vi "PicoErrorHandler.vi"(1 "error in":errorcluster) -> (0 "error out":errorcluster)   [LabVIEW 2020]
doc: "This VI takes an error cluster and if an error has occurred, displays a message box indicating the source of the error and the status code returned by the driver."
uses:
  DialogType.ctl
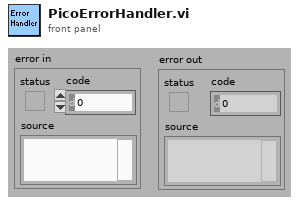
[diagram p1: front panel]
types:
  T1 = typedef "DialogType.ctl" = u16
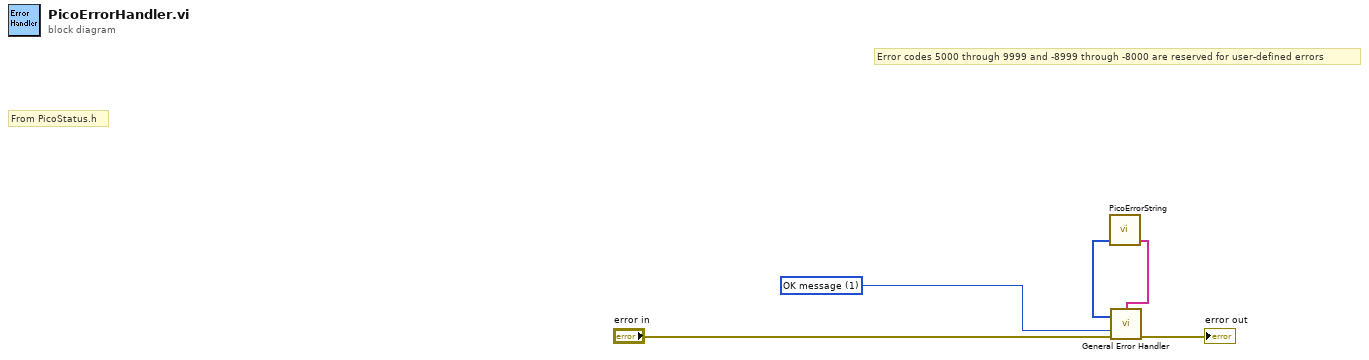
[diagram p0: block diagram]
diagram:
  w5 = T1 1 items=["no dialog", "OK message", "continue or stop message", "OK message + warnings", "continue/stop + warnings"] ("type of dialog (OK msg:1)")
  # "Error codes 5000 through 9999 and -8999 through -8000 are reserved for user-defined errors"
  # "From PicoStatus.h"
  n1 = call "PicoErrorString.vi"() -> ("[user-defined descriptions]"=w1:string[], "[user-defined codes]"=w2:u32[])  [unwired: 3 in, 1 out]
  n2 = call "General Error Handler.vi"("[user-defined codes]"=w2, "[user-defined descriptions]"=w1, "type of dialog (OK msg:1)"=w5, "error in (no error)"="error in") -> ("error out"=→"error out":errorcluster)  [unwired: 7 in, 4 out]
